vi "9205 Read.vi"(8 "error in":errorcluster, 11 "Module Config Selector":i16) -> (0 "error out":errorcluster, 3 "Data Array":sgl[](array[numeric]))   [LabVIEW 2015]
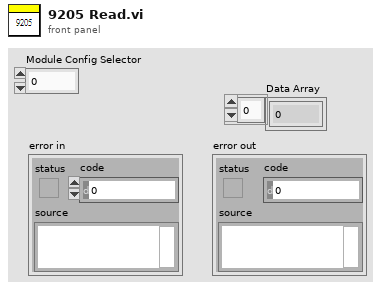
[diagram p1: front panel]
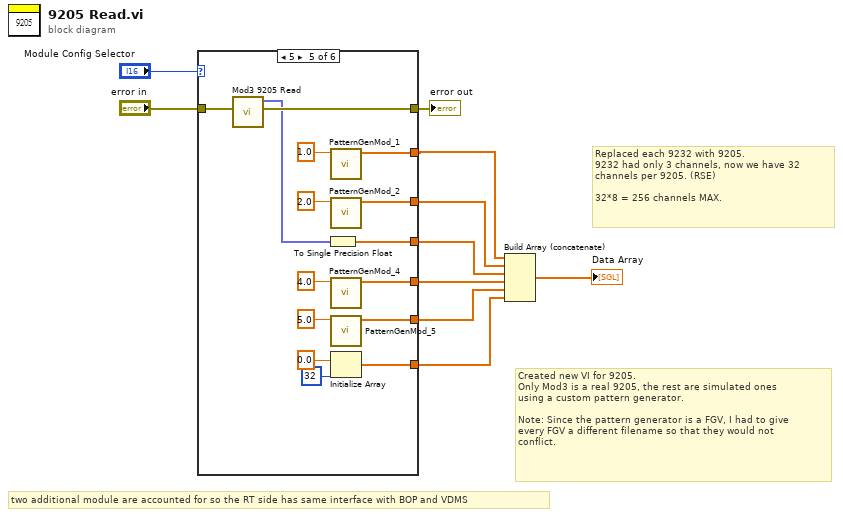
[diagram p0: block diagram]
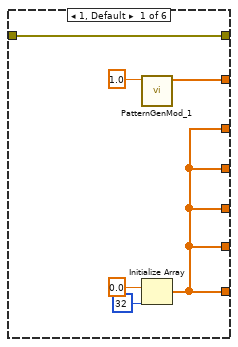
[diagram p2: hidden frame]
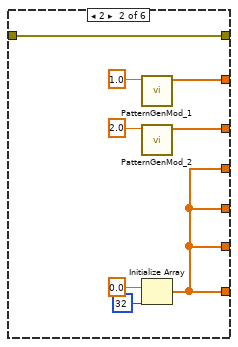
[diagram p3: hidden frame]
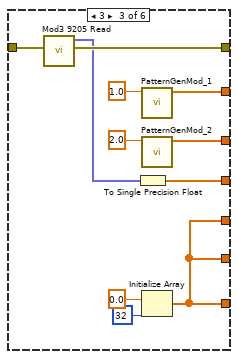
[diagram p4: hidden frame]
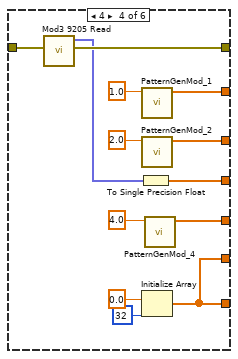
[diagram p5: hidden frame]
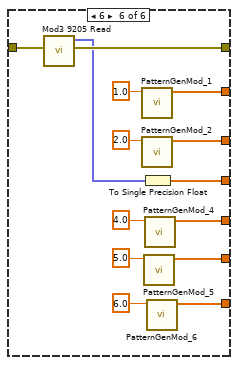
[diagram p6: hidden frame]
diagram:
  # "Replaced each 9232 with 9205.\n9232 had only 3 channels, now we have 32\nchannels per 9205. (RSE)\n\n32*8 = 256 channels MAX."
  # "Created new VI for 9205.\nOnly Mod3 is a real 9205, the rest are simulated ones\nusing a custom pattern generator.\n\nNote: Since the pattern generator is a FGV, I had to give\nevery FGV a different filename so that they would not\nconflict."
  # "two additional module are accounted for so the RT side has same interface with BOP and VDMS"
  n1 = case shown="5" "Module Config Selector" {
    tunnel: "error in" -> [w12 w17 w35 w48 w63 w77]
    tunnel: [w12 w17 w34 w47 w62 w76] -> w9
    tunnel: [w11 w18 w25 w36 w49 w64] -> w6
    tunnel: [w16 w24 w33 w45 w60 w74] -> w5
    tunnel: [w11 w22 w31 w43 w58 w72] -> w4
    tunnel: [w11 w18 w27 w41 w56 w70] -> w3
    tunnel: [w11 w18 w27 w37 w54 w68] -> w2
    tunnel: [w11 w18 w27 w37 w50 w66] -> w1
    frame 1, Default {
      n2 = call "PatternGenMod_1.vi"("DC offset"=sgl 1.0) -> ("array"=w16:sgl[])  [unwired: 10 in]
      n3 = Initialize Array(sgl 0.0 ("element"), 32 ("dimension size")) -> (w11:sgl[])
    }
    frame 2 {
      n4 = call "PatternGenMod_1.vi"("DC offset"=sgl 1.0) -> ("array"=w24:sgl[])  [unwired: 10 in]
      n5 = call "PatternGenMod_2.vi"("DC offset"=sgl 2.0) -> ("array"=w22:sgl[])  [unwired: 10 in]
      n6 = Initialize Array(sgl 0.0 ("element"), 32 ("dimension size")) -> (w18:sgl[])
    }
    frame 3 {
      n7 = call "Mod3 9205 Read.vi"("error in"=w35) -> ("error out"=w34:errorcluster, "data out"=w26:fxp<+/-,26,5>[])  [unwired: 9 in]
      n8 = To Single Precision Float(number=w26) -> (single precision float=w25:sgl[])
      n9 = call "PatternGenMod_1.vi"("DC offset"=sgl 1.0) -> ("array"=w33:sgl[])  [unwired: 10 in]
      n10 = call "PatternGenMod_2.vi"("DC offset"=sgl 2.0) -> ("array"=w31:sgl[])  [unwired: 10 in]
      n11 = Initialize Array(sgl 0.0 ("element"), 32 ("dimension size")) -> (w27:sgl[])
    }
    frame 4 {
      n12 = call "Mod3 9205 Read.vi"("error in"=w48) -> ("error out"=w47:errorcluster, "data out"=w46:fxp<+/-,26,5>[])  [unwired: 9 in]
      n13 = To Single Precision Float(number=w46) -> (single precision float=w36:sgl[])
      n14 = call "PatternGenMod_1.vi"("DC offset"=sgl 1.0) -> ("array"=w45:sgl[])  [unwired: 10 in]
      n15 = call "PatternGenMod_2.vi"("DC offset"=sgl 2.0) -> ("array"=w43:sgl[])  [unwired: 10 in]
      n16 = Initialize Array(sgl 0.0 ("element"), 32 ("dimension size")) -> (w37:sgl[])
      n17 = call "PatternGenMod_4.vi"("DC offset"=sgl 4.0) -> ("array"=w41:sgl[])  [unwired: 10 in]
    }
    frame 5 {
      n18 = call "Mod3 9205 Read.vi"("error in"=w63) -> ("error out"=w62:errorcluster, "data out"=w61:fxp<+/-,26,5>[])  [unwired: 9 in]
      n19 = To Single Precision Float(number=w61) -> (single precision float=w49:sgl[])
      n20 = call "PatternGenMod_1.vi"("DC offset"=sgl 1.0) -> ("array"=w60:sgl[])  [unwired: 10 in]
      n21 = call "PatternGenMod_2.vi"("DC offset"=sgl 2.0) -> ("array"=w58:sgl[])  [unwired: 10 in]
      n22 = call "PatternGenMod_4.vi"("DC offset"=sgl 4.0) -> ("array"=w56:sgl[])  [unwired: 10 in]
      n23 = call "PatternGenMod_5.vi"("DC offset"=sgl 5.0) -> ("array"=w54:sgl[])  [unwired: 10 in]
      n24 = Initialize Array(sgl 0.0 ("element"), 32 ("dimension size")) -> (w50:sgl[])
    }
    frame 6 {
      n25 = call "Mod3 9205 Read.vi"("error in"=w77) -> ("error out"=w76:errorcluster, "data out"=w75:fxp<+/-,26,5>[])  [unwired: 9 in]
      n26 = call "PatternGenMod_1.vi"("DC offset"=sgl 1.0) -> ("array"=w74:sgl[])  [unwired: 10 in]
      n27 = call "PatternGenMod_2.vi"("DC offset"=sgl 2.0) -> ("array"=w72:sgl[])  [unwired: 10 in]
      n28 = To Single Precision Float(number=w75) -> (single precision float=w64:sgl[])
      n29 = call "PatternGenMod_5.vi"("DC offset"=sgl 5.0) -> ("array"=w68:sgl[])  [unwired: 10 in]
      n30 = call "PatternGenMod_4.vi"("DC offset"=sgl 4.0) -> ("array"=w70:sgl[])  [unwired: 10 in]
      n31 = call "PatternGenMod_6.vi"("DC offset"=sgl 6.0) -> ("array"=w66:sgl[])  [unwired: 10 in]
    }
  }
  "error out" <- w9
  n32 = Build Array (concatenate)(w5, w4, w6, w3, w2, w1) -> (→"Data Array":sgl[])
